vi "Delay with error.vi"(6 "milliseconds to wait":u32, 8 "error in (no error)":errorcluster) -> (0 "error out":errorcluster)   [LabVIEW 2018]
doc: "Delay function with error in/out\n(like in openG lib)"
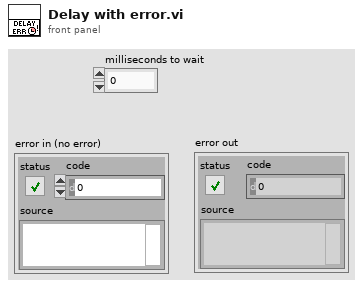
[diagram p1: front panel]
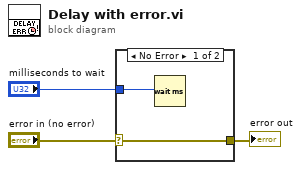
[diagram p0: block diagram]
diagram:
  n1 = case shown="No Error" "error in (no error)" {
    selector: "error in (no error)" -> [w5 w6]
    tunnel: [w5 w6] -> w2
    tunnel: "milliseconds to wait" -> [w4 _]
    frame No Error {
      n2 = Wait (ms)(milliseconds to wait=w4) -> ()  [unwired: 1 out]
    }
    frame Error {
    }
  }
  "error out" <- w2
